vi "amp_onoff.vi"(1 "error in":errorcluster, 2 "amp_onoff":bool, 3 "AMP address":tag="Dev1/port0/line0") -> (0 "error out":errorcluster)   [LabVIEW 2019]
uses:
  <vilib>/DAQmx/write.llb/DAQmx Write (Digital Bool 1Line 1Point).vi
  <vilib>/DAQmx/create/channels.llb/DAQmx Create Channel (DO-Digital Output).vi
  <vilib>/DAQmx/miscellaneous.llb/DAQmx Fill In Error Info.vi
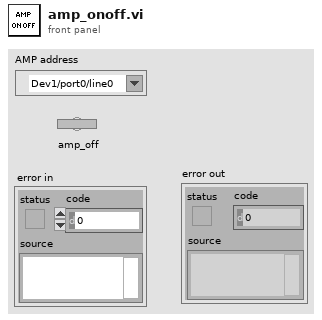
[diagram p1: front panel]
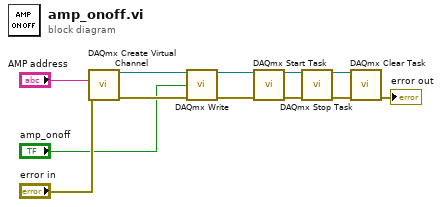
[diagram p0: block diagram]
diagram:
  n1 = call-poly <vilib>:"DAQmx Create Virtual Channel.vi"("lines"="AMP address", "error in"="error in") -> ("task out"=w8:refnum<k21>, "error out"=w6:errorcluster)  [unwired: 12 in]
  n2 = call-poly <vilib>:"DAQmx Write.vi"("task/channels in"=w8, "data"="amp_onoff", "error in"=w6) -> ("task out"=w11:refnum<k21>, "error out"=w5:errorcluster)  [unwired: 10 in, 1 out]
  n3 = call <vilib>:"DAQmx Start Task.vi"("task/channels in"=w11, "error in"=w5) -> ("task out"=w9:refnum<k21>, "error out"=w4:errorcluster)  [unwired: 12 in]
  n4 = call <vilib>:"DAQmx Stop Task.vi"("task/channels in"=w9, "error in"=w4) -> ("task out"=w10:refnum<k21>, "error out"=w3:errorcluster)  [unwired: 12 in]
  n5 = call <vilib>:"DAQmx Clear Task.vi"("task in"=w10, "error in"=w3) -> ("error out"=→"error out":errorcluster)  [unwired: 13 in]
